vi "TPNormalRun.vi"(0 "Voltage SP":dbl, 1 "COM-Port":bool, 2 "Current SP":dbl=5000.0, 3 "Power SP":dbl=150.0, 4 "reference":refnum<visa-resource-name>, 5 "Control Byte":string) -> (6 "Voltage Out":dbl, 7 "Current Out":dbl, 8 "Power Out":dbl)   [LabVIEW 2017]
panel:
  out "error out":errorcluster
  out "Output String":string
  out "Virtual Power":dbl
  out "Virtual Current":dbl
  out "Virtual Voltage":dbl
  out "Number of Bytes\nRecieved":u32
  out "Bytes sent":u32
  out "Command sent":string
  # "Mains Relays: (1)On (0)Off\nPower: Off(0), On(1)\nReset arc counters: 1\n-\nAnalog: (1)\nPC Controls TruPlasma(1), Monitoring only(0)\nProfibus control(1)\nDisplay control(1)"
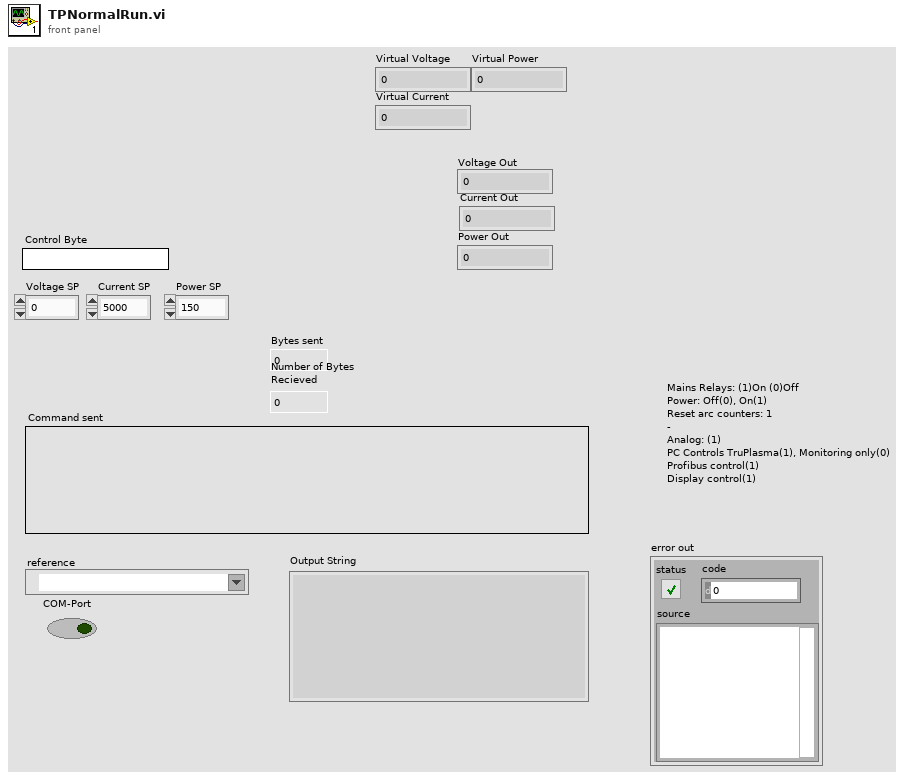
[diagram p1: front panel]
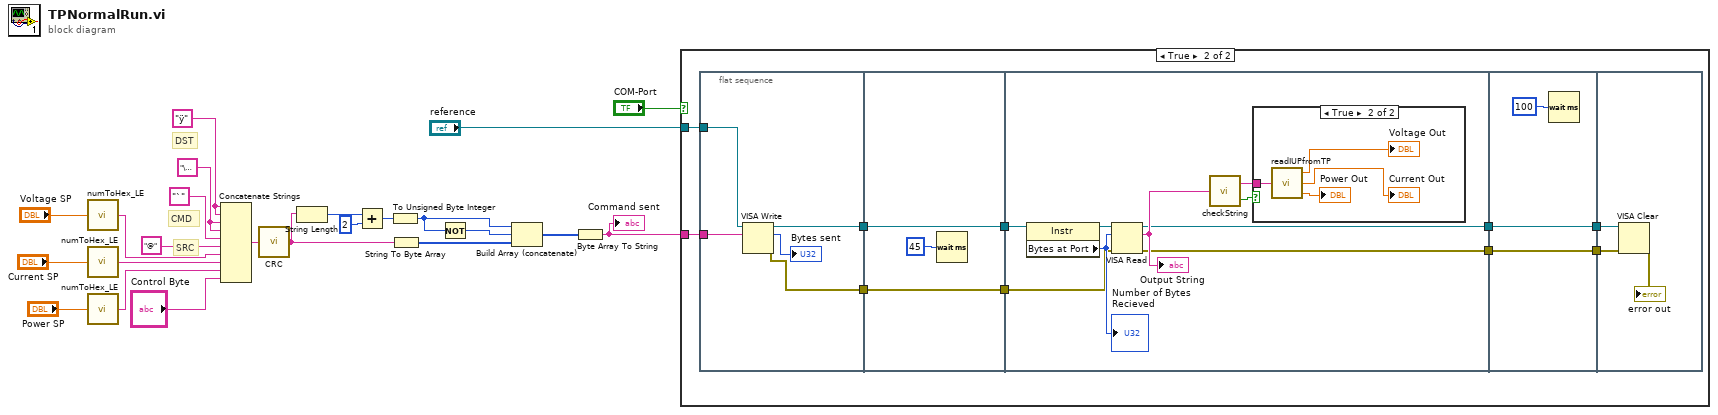
[diagram p0: block diagram]
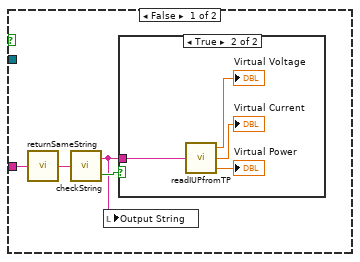
[diagram p2: hidden frame]
diagram:
  w22 = "\u0000" ("SRC")
  w23 = "ÿ" ("DST")
  # "CMD"
  # "SRC"
  # "DST"
  n1 = call "numToHex_LE.vi"("Numeric"="Voltage SP") -> ("string"=w9:string)
  n2 = call "numToHex_LE.vi"("Numeric"="Current SP") -> ("string"=w8:string)
  n3 = call "numToHex_LE.vi"("Numeric"="Power SP") -> ("string"=w7:string)
  n4 = Concatenate Strings(w23, w23, w22, w22, "`" ("CMD_H"), "@" ("CMD_L"), w9, w8, w7, "Control Byte") -> (w11:string)
  n5 = call "CRC.vi"("Input String"=w11) -> ("String w/ CRC"=w17:string)
  n6 = String Length(string=w17) -> (length=w19:i32)
  n7 = Add(x=w19, y=2) -> (x+y=w14:i32)
  n8 = To Unsigned Byte Integer(number=w14) -> (unsigned 8bit integer=w13:u8)
  n9 = String To Byte Array(string=w17) -> (unsigned byte array=w16:u8[])
  n10 = Not(x=w13) -> (.not. x?=w12:u8)
  n11 = Build Array (concatenate)(w13, w12, w16) -> (w15:u8[])
  n12 = Byte Array To String(unsigned byte array=w15) -> (string=w2:string)
  "Command sent" <- w2
  n13 = case shown="True" "COM-Port" {
    tunnel: "reference" -> [_ w39]
    tunnel: w2 -> [w26 w38]
    frame False {
      n14 = call "returnSameString.vi"("String"=w26) -> ("substring"=w25:string)
      n15 = call "checkString.vi"("String"=w25) -> ("String Out"=w24:string, "TRUE OR FALSE"=w27:bool)
      n16 = local write "Output String"(w24) -> ()
      n17 = case shown="True" w27 {
        tunnel: w24 -> [_ w28]
        frame False {
        }
        frame True {
          n18 = call "readIUPfromTP.vi"("HEX String to Decode"=w28) -> ("Numeric"=→"Virtual Voltage":dbl, "Numeric 2"=→"Virtual Current":dbl, "Numeric 3"=→"Virtual Power":dbl)
        }
      }
    }
    frame True {
      n19 = flat-sequence {
        tunnel: [w46] -> w41
        tunnel: w39 -> [w44]
        tunnel: w38 -> [w43]
        tunnel: [w42] -> w34
        tunnel: w41 -> [w49]
        tunnel: [w49] -> w40
        tunnel: [w47] -> w35
        tunnel: w34 -> [w47]
        tunnel: w40 -> [w56]
        tunnel: [w52] -> w37
        tunnel: w35 -> [w51]
        tunnel: [w50] -> w32
        tunnel: w37 -> [w65]
        tunnel: [w65] -> w36
        tunnel: [w63] -> w33
        tunnel: w32 -> [w63]
        tunnel: w36 -> [w68]
        tunnel: w33 -> [w67]
        frame #0 {
          n20 = VISA Write(VISA resource name=w44, write buffer=w43) -> (VISA resource name out=w46:refnum<visa-resource-name>, return count=→"Bytes sent":u32, error out=w42:errorcluster)  [unwired: 1 in]
        }
        frame #1 {
          n21 = Wait (ms)(milliseconds to wait=u32 45) -> ()  [unwired: 1 out]
        }
        frame #2 {
          n22 = property class="Instr"(reference=w56) -> (reference out=w58:refnum<visa-resource-name>, "Bytes at Port"=w57:u32)  [unwired: 1 in, 1 out]
          "Number of Bytes\nRecieved" <- w57
          n23 = VISA Read(VISA resource name=w58, byte count=w57, error in (no error)=w51) -> (VISA resource name out=w52:refnum<visa-resource-name>, read buffer=w55:string, error out=w50:errorcluster)  [unwired: 1 out]
          "Output String" <- w55
          n24 = call "checkString.vi"("String"=w55) -> ("String Out"=w54:string, "TRUE OR FALSE"=w53:bool)
          n25 = case shown="True" w53 {
            tunnel: w54 -> [_ w59]
            frame False {
            }
            frame True {
              n26 = call "readIUPfromTP.vi"("HEX String to Decode"=w59) -> ("Numeric"=→"Voltage Out":dbl, "Numeric 2"=→"Current Out":dbl, "Numeric 3"=→"Power Out":dbl)
            }
          }
        }
        frame #3 {
          n27 = Wait (ms)(milliseconds to wait=u32 100) -> ()  [unwired: 1 out]
        }
        frame #4 {
          n28 = VISA Clear(VISA resource name=w68, error in (no error)=w67) -> (error out=→"error out":errorcluster)  [unwired: 1 out]
        }
      }
    }
  }
